vi "Remove Observer.vi"(8 "error in (no error)":errorcluster, 10 "Observer":refnum<class "Observer.lvclass">, 11 "Observable in":refnum<class "Observable.lvclass">) -> (0 "error out":errorcluster, 3 "Observable out":refnum<class "Observable.lvclass">)   [LabVIEW 2011, in "Observable.lvclass"]
uses:
  Observable.lvclass
  Observer/Observer.lvclass
  Observable.lvclass/Observable.ctl
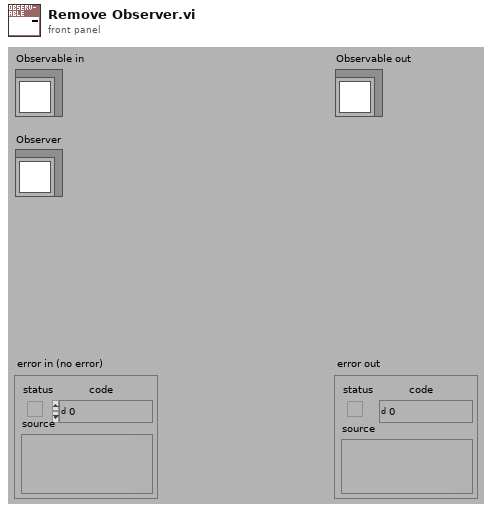
[diagram p1: front panel]
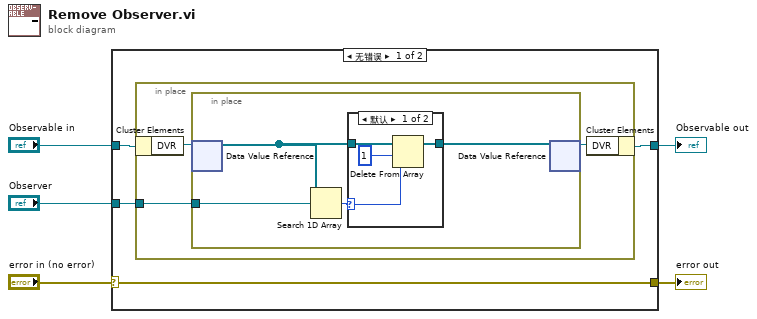
[diagram p0: block diagram]
diagram:
  n1 = case shown="无错误" "error in (no error)" {
    selector: "error in (no error)" -> [w6 w23]
    tunnel: "Observable in" -> [w9 w22]
    tunnel: [w8 w22] -> w4
    tunnel: "Observer" -> [w7 _]
    tunnel: [w6 w23] -> w1
    frame No Error {
      n2 = in-place {
        in-place-border: w7 -> [w10]
        n3 = in-place-cluster #1(w9) -> ("DVR"=w12:refnum<data-value>)
        n4 = in-place {
          in-place-border: w10 -> [w16]
          n5 = in-place-dvr #2(w12) -> (w14:refnum<class "Observer.lvclass">[])  [unwired: 1 out]
          n6 = Search 1D Array(1D array=w14, element=w16) -> (index of element=w15:i32)  [unwired: 1 in]
          n7 = case shown="默认" w15 {
            selector: w15 -> [w19 _]
            tunnel: [w20 w21] -> w13
            tunnel: w14 -> [w17 w21]
            frame Default {
              n8 = Delete From Array(array=w17, length=1, index=w19) -> (array with subset deleted=w20:refnum<class "Observer.lvclass">[])  [unwired: 1 out]
            }
            frame -1 {
            }
          }
          n9 = in-place-dvr #2(w13) -> (w11:refnum<data-value>)  [unwired: 1 out]
        }
        n10 = in-place-cluster #1("DVR"=w11) -> (w8:refnum<class "Observable.lvclass">)
      }
    }
    frame Error {
    }
  }
  "Observable out" <- w4
  "error out" <- w1
